vi "Vision.vi"(6 "Filter Values":T6(array[cluster]) {"Measurement Parameter" items=["Center of Mass X", "Center of Mass Y", "First Pixel X", "First Pixel Y", "Bounding Rect Left", "Bounding Rect Top", "Bounding Rect Right", "Bounding Rect Bottom", "Max Feret Diameter Start X", "Max Feret Diameter Start Y", "Max Feret Diameter End X", "Max Feret Diameter End Y", "Max Horiz. Segment Length Left", "Max Horiz. Segment Length Right", "Max Horiz. Segment Length Row", "-", "Bounding Rect Width", "Bounding Rect Height", "Bounding Rect Diagonal", "Perimeter", "Convex Hull Perimeter", "Holes' Perimeter", "Max Feret Diameter", "Equivalent Ellipse Major Axis", "Equivalent Ellipse Minor Axis", "Equivalent Ellipse Minor Axis (Feret)", "Equivalent Rect Long Side", "Equivalent Rect Short Side", "Equivalent Rect Diagonal", "Equivalent Rect Short Side (Feret)", "Average Horiz. Segment Length", "Average Vert. Segment Length", "Hydraulic Radius", "Waddel Disk Diameter", "-", "Area", "Holes' Area", "Particle & Holes' Area", "Convex Hull Area", "Image Area", "-", "Number of Holes", "Number of Horiz. Segments", "Number of Vert. Segments", "-", "Orientation", "Max Feret Diameter Orientation", "-", "% Area/Image Area", "% Area/(Particle & Holes' Area)", "Ratio of Equivalent Ellipse Axes", "Ratio of Equivalent Rect Sides", "-", "Elongation Factor", "Compactness Factor", "Heywood Circularity Factor", "Type Factor", "-", "Sum X", "Sum Y", "Sum XX", "Sum XY", "Sum YY", "Sum XXX", "Sum XXY", "Sum XYY", "Sum YYY", "-", "Moment of Inertia XX", "Moment of Inertia XY", "Moment of Inertia YY", "Moment of Inertia XXX", "Moment of Inertia XXY", "Moment of Inertia XYY", "Moment of Inertia YYY", "Norm. Moment of Inertia XX", "Norm. Moment of Inertia XY", "Norm. Moment of Inertia YY", "Norm. Moment of Inertia XXX", "Norm. Moment of Inertia XXY", "Norm. Moment of Inertia XYY", "Norm. Moment of Inertia YYY", "Hu Moment 1", "Hu Moment 2", "Hu Moment 3", "Hu Moment 4", "Hu Moment 5", "Hu Moment 6", "Hu Moment 7"]; "Range Lower Value" format="%.2f"; "Range Upper Value" format="%.2f"}, 8 "Distance Inputs":T2, 9 "RGB Filters":T3={"Red"={"Lower value"=0, "Upper value"=255}, "Green"={"Lower value"=0, "Upper value"=255}, "Blue"={"Lower value"=0, "Upper value"=255}}, 10 "Switches":cluster{"Convex":bool, "Particle Filter":bool}, 11 "RGB Input":T4) -> (0 "Particle Reports":T1 {"Particle Reports (Pixel)"."Orientation" format="%.2f"; "Particle Reports (Pixel)"."Dimensions"."Height" format="%.2f"; "Particle Reports (Pixel)"."Dimensions"."Width" format="%.2f"; "Particle Reports (Pixel)"."Center of Mass"."Y" format="%.2f"; "Particle Reports (Pixel)"."Center of Mass"."X" format="%.2f"; "Particle Reports (Pixel)"."Bounding Rect"."Bottom" format="%.2f"; "Particle Reports (Pixel)"."Bounding Rect"."Right" format="%.2f"; "Particle Reports (Pixel)"."Bounding Rect"."Top" format="%.2f"; "Particle Reports (Pixel)"."Bounding Rect"."Left" format="%.2f"; "Particle Reports (Pixel)"."Number of Holes" format="%.2f"; "Particle Reports (Pixel)"."Area" format="%.2f"; "Particle Reports (Real-World)"."Orientation" format="%.2f"; "Particle Reports (Real-World)"."Dimensions"."Height" format="%.2f"; "Particle Reports (Real-World)"."Dimensions"."Width" format="%.2f"; "Particle Reports (Real-World)"."Center of Mass"."Y" format="%.2f"; "Particle Reports (Real-World)"."Center of Mass"."X" format="%.2f"; "Particle Reports (Real-World)"."Bounding Rect"."Bottom" format="%.2f"; "Particle Reports (Real-World)"."Bounding Rect"."Right" format="%.2f"; "Particle Reports (Real-World)"."Bounding Rect"."Top" format="%.2f"; "Particle Reports (Real-World)"."Bounding Rect"."Left" format="%.2f"; "Particle Reports (Real-World)"."Number of Holes" format="%.2f"; "Particle Reports (Real-World)"."Area" format="%.2f"}, 1 "Distance":dbl, 2 "Binary Output":T4, 3 "RGB Output":T4)   [LabVIEW 2015]
uses:
  <vilib>/vision/Image Controls.llb/IMAQ Image.ctl
  <vilib>/vision/NI_Vision_Development_Module.lvlib
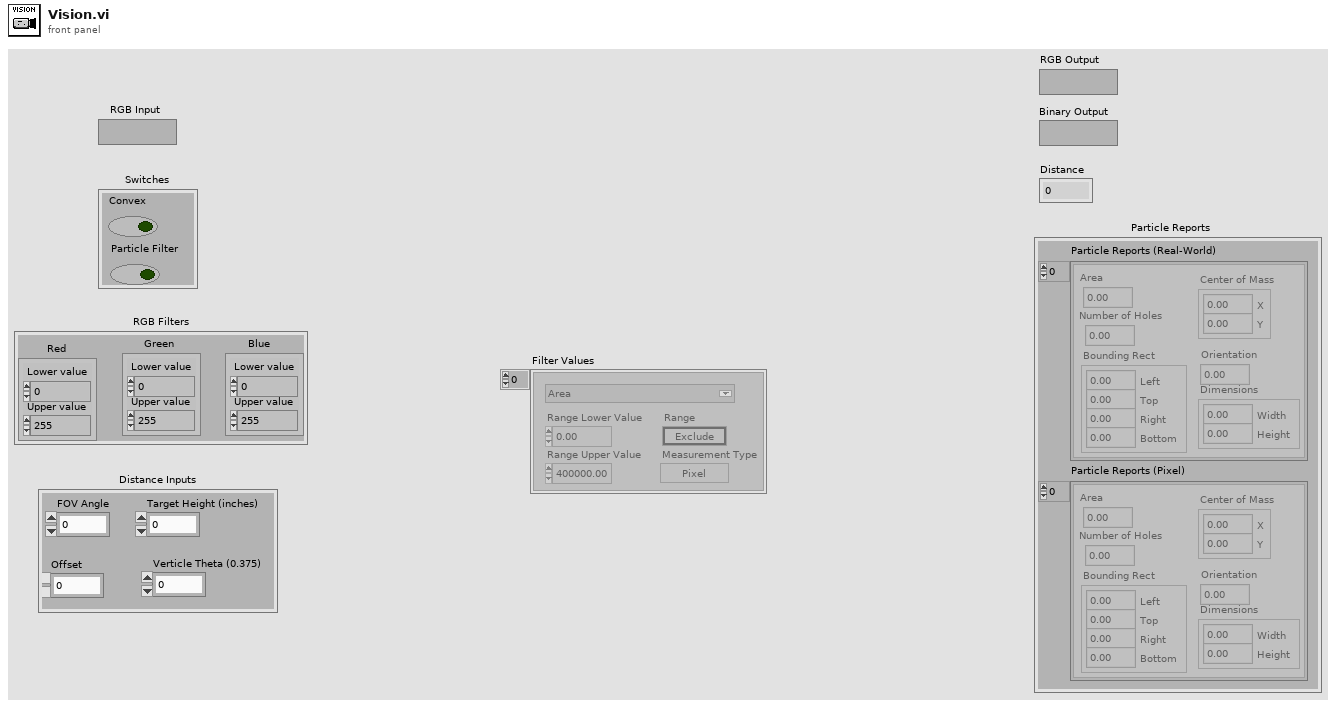
[diagram p1: front panel]
types:
  T1 = cluster{"Particle Reports (Real-World)  ":cluster{"Area":dbl, "Number of Holes":dbl, "Bounding Rect":cluster{"Left":dbl, "Top":dbl, "Right":dbl, "Bottom":dbl}, "Center of Mass":cluster{"X":dbl, "Y":dbl}, "Orientation":dbl, "Dimensions":cluster{"Width":dbl, "Height":dbl}}[], "Particle Reports (Pixel)":cluster{"Area":dbl, "Number of Holes":dbl, "Bounding Rect":cluster{"Left":dbl, "Top":dbl, "Right":dbl, "Bottom":dbl}, "Center of Mass":cluster{"X":dbl, "Y":dbl}, "Orientation":dbl, "Dimensions":cluster{"Width":dbl, "Height":dbl}}[]}
  T2 = cluster{"FOV Angle":dbl, "Target Height (inches)":dbl, "Offset":dbl, "Verticle Theta (0.375)":dbl}
  T3 = cluster{"Red":cluster{"Lower value":i32, "Upper value":i32}, "Green":cluster{"Lower value":i32, "Upper value":i32}, "Blue":cluster{"Lower value":i32, "Upper value":i32}}
  T4 = typedef "IMAQ Image.ctl" = refnum<image>
  T5 = typedef "Particle Parameters" = i32
  T6 = cluster{"Measurement Parameter":T5, "Range Lower Value":dbl, "Range Upper Value":dbl, "Range":bool, "Measurement Type":bool}[]
  T7 = typedef "Image Type" = u32
  T8 = cluster{"Area":dbl, "Number of Holes":dbl, "Bounding Rect":cluster{"Left":dbl, "Top":dbl, "Right":dbl, "Bottom":dbl}, "Center of Mass":cluster{"X":dbl, "Y":dbl}, "Orientation":dbl, "Dimensions":cluster{"Width":dbl, "Height":dbl}}[]
  T9 = cluster{"Particle Reports (Real-World)  ":cluster{"Area":dbl, "Number of Holes":dbl, "Bounding Rect":cluster{"Left":dbl, "Top":dbl, "Right":dbl, "Bottom":dbl}, "Center of Mass":cluster{"X":dbl, "Y":dbl}, "Orientation":dbl, "Dimensions":cluster{"Width":dbl, "Height":dbl}}[], "Particle Reports (Pixels)":cluster{"Area":dbl, "Number of Holes":dbl, "Bounding Rect":cluster{"Left":dbl, "Top":dbl, "Right":dbl, "Bottom":dbl}, "Center of Mass":cluster{"X":dbl, "Y":dbl}, "Orientation":dbl, "Dimensions":cluster{"Width":dbl, "Height":dbl}}[]}
  T10 = cluster{"Area":dbl, "Number of Holes":dbl, "Bounding Rect":cluster{"Left":dbl, "Top":dbl, "Right":dbl, "Bottom":dbl}, "Center of Mass":cluster{"X":dbl, "Y":dbl}, "Orientation":dbl, "Dimensions":cluster{"Width":dbl, "Height":dbl}}
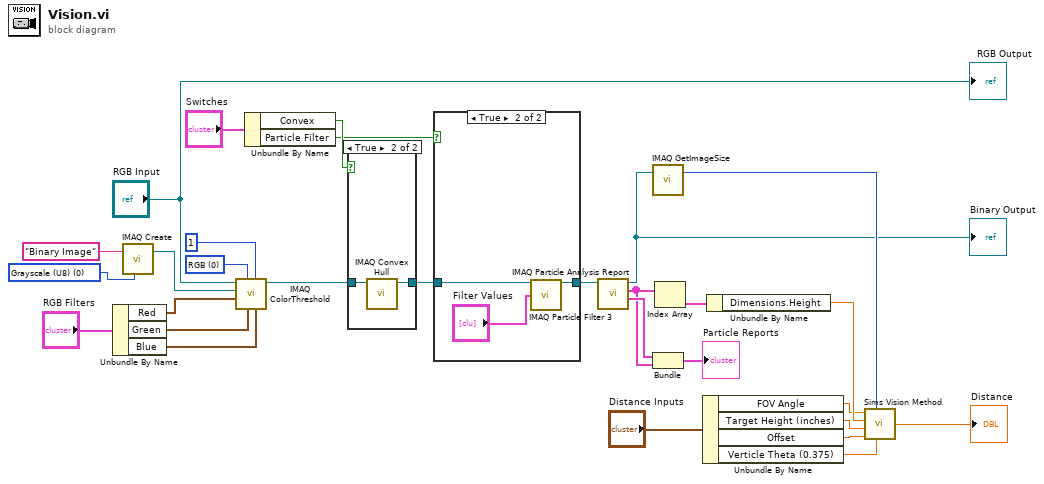
[diagram p0: block diagram]
diagram:
  w25 = T7 0 items=["Grayscale (U8)", "Grayscale (I16)", "Grayscale (SGL)", "Complex (CSG)", "RGB (U32)", "HSL (U32)", "RGB (U64)", "Grayscale (U16)"] ("Image Type")
  w29 = u16 0 items=["RGB", "HSL", "HSV", "HSI"] ("Color Mode")
  n1 = Unbundle By Name("RGB Filters") -> ("Red"=w16:cluster{"Lower value":i32, "Upper value":i32}, "Green"=w15:cluster{"Lower value":i32, "Upper value":i32}, "Blue"=w14:cluster{"Lower value":i32, "Upper value":i32})
  n2 = call "IMAQ Create"("Image Name"="Binary Image", "Image Type"=w25) -> ("New Image"=w24:T4)  [unwired: 3 in, 1 out]
  n3 = call "IMAQ ColorThreshold"("Blue or Luma or Val or Inten Range"=w14, "Replace Value"=1, "Green or Sat Range"=w15, "Color Mode"=w29, "Red or Hue Range"=w16, "Image Dst"=w24, "Image Src"="RGB Input") -> ("Image Dst Out"=w23:T4)  [unwired: 3 in, 1 out]
  n4 = Unbundle By Name("Switches") -> ("Convex"=w12:bool, "Particle Filter"=w11:bool)
  n5 = case shown="True" w12 {
    tunnel: w23 -> [w30 w32]
    tunnel: [w30 w31] -> w22
    frame False {
    }
    frame True {
      n6 = call "IMAQ Convex Hull"("Image Src"=w32) -> ("Image Dst Out"=w31:T4)  [unwired: 9 in, 1 out]
    }
  }
  n7 = case shown="True" w11 {
    tunnel: w22 -> [w33 w36]
    tunnel: [w33 w35] -> w21
    frame False {
    }
    frame True {
      n8 = call "IMAQ Particle Filter 3"("Image Src"=w36, "Selection Values"="Filter Values") -> ("Image Dst Out"=w35:T4)  [unwired: 11 in, 2 out]
    }
  }
  n9 = call "IMAQ Particle Analysis Report"("Image"=w21) -> ("Particle Reports (Real-World)"=w2:T8, "Particle Reports (Pixels)"=w1:T8, "Image Out (duplicate)"=w18:T4)  [unwired: 5 in, 3 out]
  "Binary Output" <- w18
  n10 = call "IMAQ GetImageSize"("Image"=w18) -> ("Y Resolution"=w19:i32)  [unwired: 3 in, 2 out]
  n11 = Bundle("Particle Reports (Real-World)"=w2, "Particle Reports (Pixels)"=w1) -> (→"Particle Reports":T9)  [unwired: 1 in]
  n12 = Index Array(array=w1) -> (element=w10:T10)  [unwired: 1 in]
  n13 = Unbundle By Name("Distance Inputs") -> ("FOV Angle"=w7:dbl, "Target Height (inches)"=w6:dbl, "Offset"=w5:dbl, "Verticle Theta (0.375)"=w4:dbl)
  n14 = Unbundle By Name(w10) -> ("Dimensions.Height"=w9:dbl)
  n15 = call "Sims Vision Method.vi"("Vert Theta (0.375)"=w4, "Image Hight In Pixels"=w19, "Offset"=w5, "Target Height In Inches"=w6, "Target Hight In Pixels"=w9, "FOV Angle"=w7) -> ("Distance"=→"Distance":dbl)
  "RGB Output" <- "RGB Input"
